vi "Unpack Listbox Edit Cell.vi"(11 "ListboxEditCellMsg":refnum<class "ListboxEditCellMsg.lvclass">) -> (0 "String":string, 1 "Time":u32, 2 "Control Label":string, 3 "CtlRef":refnum<vi>, 4 "Coords":T1)   [LabVIEW 2015, in "ActorEvents.lvlib" / "ListboxEditCellMsg.lvclass"]
doc: "<License>\nCopyright © 2017 Composed Systems, LLC | All rights reserved\nwww.composed.io\n\nAuthor: Ethan Stern <ethan.stern@composed.io>\n\nThis software is provided \"AS IS\" WITHOUT WARRANTIES, either express or implied, AND IS FOR EDUCATIONAL PURPOSES ONLY.\n</License>"
uses:
  ListboxEditCellMsg.lvclass
  <vilib>/Utility/miscctls.llb/LVRowAndColumnTypeDef.ctl
  ListboxEditCellMsg.lvclass/ListboxEditCellMsg.ctl
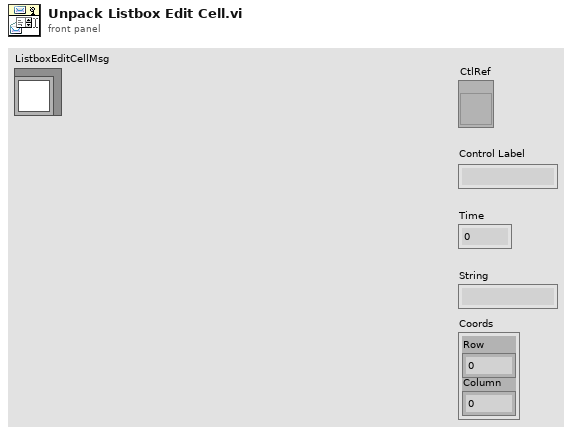
[diagram p1: front panel]
types:
  T1 = typedef "LVRowAndColumnTypeDef.ctl" = cluster{"Row":i32, "Column":i32}
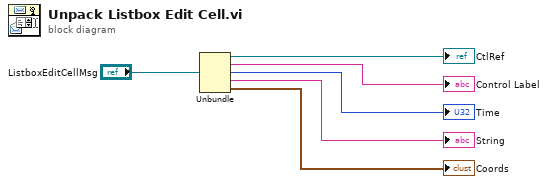
[diagram p0: block diagram]
diagram:
  n1 = Unbundle("ListboxEditCellMsg") -> (→"CtlRef":refnum<vi>, →"Control Label":string, →"Time":u32, →"String":string, →"Coords":T1)
